vi "generateModels_v4.vi"() -> ()   [LabVIEW 2016]
panel:
  out "Progress Bar":dbl(slide) max=1.0 scale=0.0..1.0
  in  "countdownStart":bool
  in  "Use Online Scan":bool
  out "error IO":errorcluster
  in  "SCAN_NO":string="0011"
  in  "Process VSCAN":bool
  in  "stop":bool
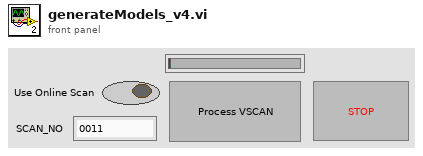
[diagram p1: front panel]
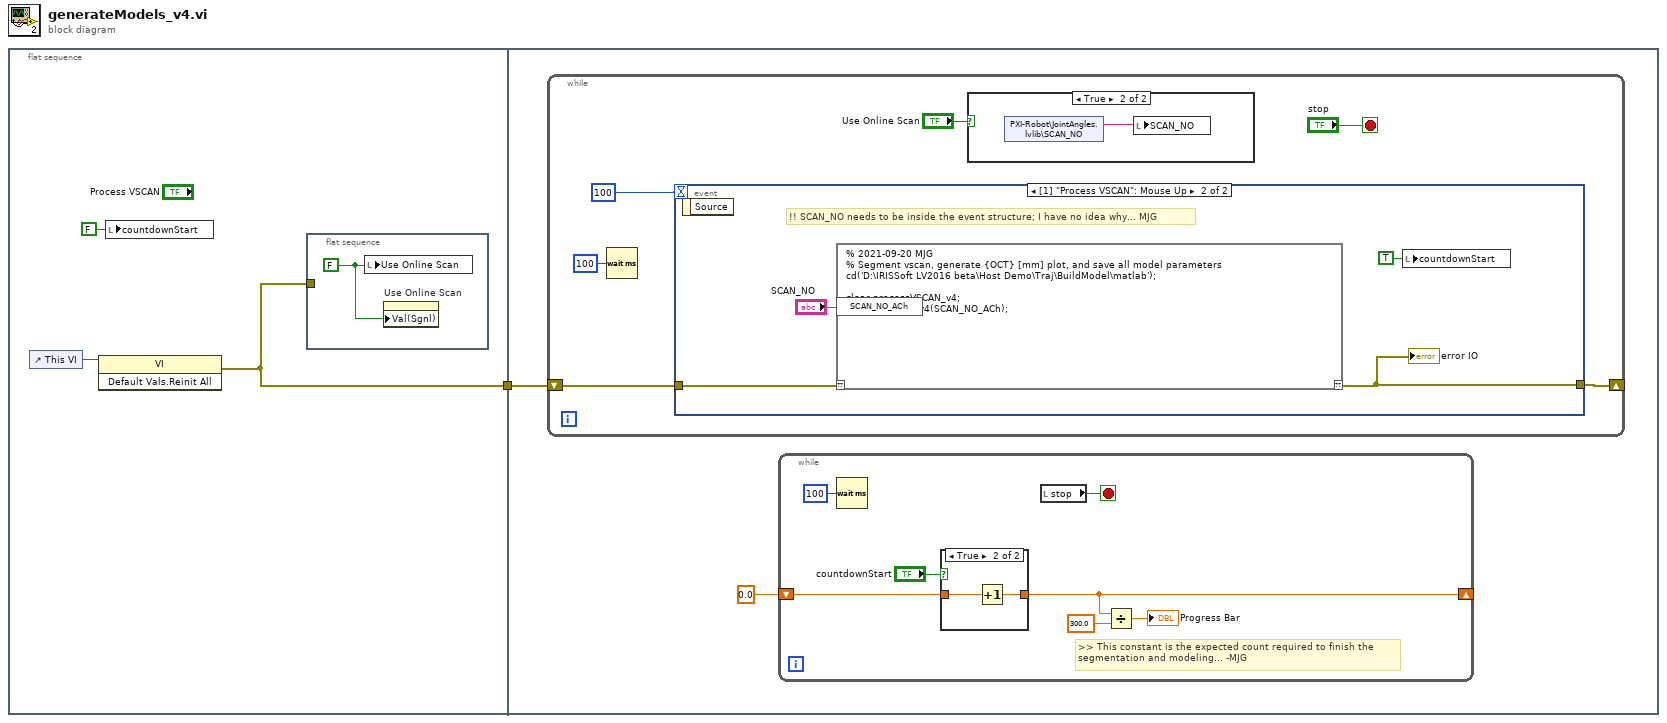
[diagram p0: block diagram]
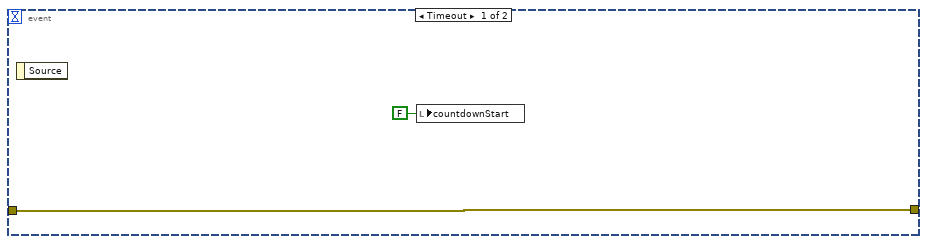
[diagram p4: hidden frame]
diagram:
  n1 = flat-sequence {
    tunnel: [w3] -> w1
    tunnel: w1 -> [w7]
    frame #0 {
      n2 = control-ref of="This VI"() -> (w4:refnum<vi>)
      n3 = invoke class="VI" method="Default Vals.Reinit All"(reference=w4) -> (error out=w3:errorcluster)  [unwired: 2 in, 2 out]
      n4 = local write "countdownStart"(FALSE ("countdownStart")) -> ()
      n5 = flat-sequence {
        tunnel: w3 -> [_]
        frame #0 {
          w5 = FALSE ("Use Online Scan")
          n6 = local write "Use Online Scan"(w5) -> ()
          n7 = property on="Use Online Scan" class="Bool (strict)"("Val(Sgnl)"=w5) -> ()  [unwired: 2 in, 2 out]
        }
      }
    }
    frame #1 {
      n8 = while {
        shift-right: [w19] -> _
        shift-left: w7 -> [w21]
        stop <- "stop" stop-if-true
        n9 = Wait (ms)(milliseconds to wait=u32 100) -> ()  [unwired: 1 out]
        n10 = event shown="[1] \"Process VSCAN\": Mouse Up" {
          selector: _ -> [_ _]
          dyn-events: _ -> [_ _]
          timeout: 100 -> [_ _]
          tunnel: [w26 w29] -> w19
          tunnel: w21 -> [w26 w30]
          event Timeout {
            # "timeout"
            n11 = event-data() -> ()  [unwired: 1 in, 1 out]
            n12 = local write "countdownStart"(FALSE ("countdownStart")) -> ()
          }
          event "Process VSCAN": Mouse Up {
            # "!! SCAN_NO needs to be inside the event structure; I have no idea why... MJG"
            # "run ML script to segment the vscan (ACh or PC)"
            n13 = event-data() -> ()  [unwired: 1 in, 1 out]
            n14 = script code="% 2021-09-20 MJG \n% Segment vscan, generate {OCT} [mm] plot, and save all model parameters\ncd('D:\\IRISSoft LV2016 beta\\Host Demo\\Traj\\BuildModel\\matlab');\n\nclear processVSCAN_v4;\nprocessVSCAN_v4(SCAN_NO_ACh);" ("Script Node")("??"=w30, "SCAN_NO_ACh"="SCAN_NO") -> ("??"=w29:errorcluster)
            "error IO" <- w29
            n15 = local write "countdownStart"(TRUE ("countdownStart")) -> ()
          }
        }
        n16 = case shown="True" "Use Online Scan" {
          frame False {
          }
          frame True {
            n17 = shared-variable "PXI-Robot\\JointAngles.lvlib\\SCAN_NO"() -> (w24:string)  [unwired: 1 in, 1 out]
            n18 = local write "SCAN_NO"(w24) -> ()
          }
        }
      }
      n19 = while {
        shift-right: [w10] -> _
        shift-left: 0.0 ("Numeric") -> [w12]
        stop <- w14 stop-if-true
        # ">> This constant is the expected count required to finish the \nsegmentation and modeling... -MJG"
        n20 = Wait (ms)(milliseconds to wait=u32 100) -> ()  [unwired: 1 out]
        n21 = case shown="True" "countdownStart" {
          tunnel: w12 -> [w15 w17]
          tunnel: [w15 w16] -> w10
          frame False {
          }
          frame True {
            n22 = Increment(x=w17) -> (x+1=w16:dbl)
          }
        }
        n23 = local read "stop"() -> (w14:bool)
        n24 = Divide(x=w10, y=300.0) -> (x/y=→"Progress Bar":dbl)
      }
    }
  }
